vi "SRV_Sensor Name to Sensor Name Enum.vi"(7 "Sensor to Edit":string, 11 "error in (no error)":errorcluster) -> (8 "Sensor View Indicator Names":T1, 10 "Sensor Index":i32, 15 "error out":errorcluster)   [LabVIEW 2009]
uses:
  SRV_Sensors Names.ctl
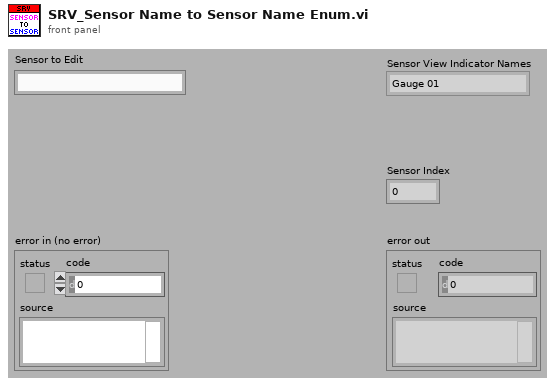
[diagram p1: front panel]
types:
  T1 = typedef "SRV_Sensors Names.ctl" = enum16{"Gauge 01", "Gauge 02", "Gauge 03", "Gauge 04", "Meter 01", "Meter 02", "Meter 03", "Meter 04", "Numeric 01", "Numeric 02", "Numeric 03", "Numeric 04", "Numeric 05", "Numeric 06", "Numeric 07", "Numeric 08", "Boolean 01", "Boolean 02", "Boolean 03", "Boolean 04", "Boolean 05", "Boolean 06", "Boolean 07", "Boolean 08", "Boolean 09", "Boolean 10", "Boolean 11", "Boolean 12", "Boolean 13", "Boolean 14", "Boolean 15", "Boolean 16", "Boolean 17", "Boolean 18", "Boolean 19", "Boolean 20", "Boolean 21", "Boolean 22", "Boolean 23", "Boolean 24", "Boolean 25", "Boolean 26", "Boolean 27", "Boolean 28", "Boolean 29", "Boolean 30", "Boolean 31", "Boolean 32"}
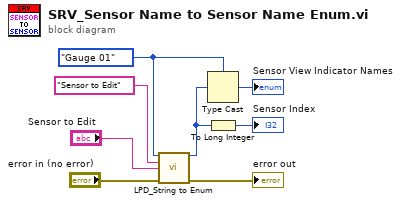
[diagram p0: block diagram]
diagram:
  w6 = SRV_Sensors_Names."Gauge 01" ("Sensor View Indicator Names")
  n1 = call "LPD_String to Enum.vi"("Variant (Enum)"=w6, "Lookup String (for error reporting)"="Sensor to Edit", "Enum Value String"="Sensor to Edit", "error in (no error)"="error in (no error)") -> ("Value (typecast back to enum)"=w2:u16, "error out"=→"error out":errorcluster)  [unwired: 10 in]
  n2 = Type Cast(type=w6, x=w2) -> (*(type *) &x=→"Sensor View Indicator Names":T1)
  n3 = To Long Integer(number=w2) -> (32bit integer=→"Sensor Index":i32)
